vi "genFnameString.vi"(1 "Idx":i32, 2 "str":string="channel0_") -> (0 "fName":string)   [LabVIEW 2015]
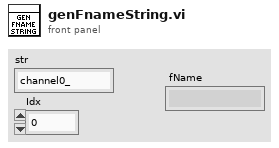
[diagram p1: front panel]
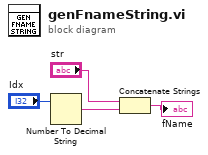
[diagram p0: block diagram]
diagram:
  n1 = Number To Decimal String(number="Idx") -> (decimal integer string=w1:string)  [unwired: 1 in]
  n2 = Concatenate Strings("str", w1) -> (→"fName":string)
